vi "PWM2 Set Frequency.vi"(7 "Precision":u16, 9 "Frequency":u32, 10 "ChannelIndex":u8, 11 "DevHandle":i32) -> (3 "function return":i32)   [LabVIEW 2010, in "usb2pwm.lvlib"]
doc: "int WINAPI PWM2_SetFrequency(int DevHandle, unsigned char ChannelIndex, unsigned int Frequency, unsigned short Precision);"
uses:
  usb2pwm.lvlib
  USB2XXX/trunk/USB2XXX/USB2XXX/vs2019/Release/USB2XXX.dll
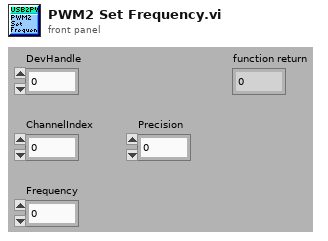
[diagram p1: front panel]
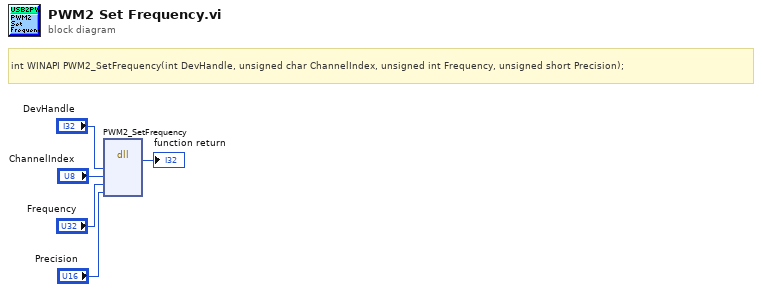
[diagram p0: block diagram]
diagram:
  # "int WINAPI PWM2_SetFrequency(int DevHandle, unsigned char ChannelIndex, unsigned int Frequency, unsigned short Precision);"
  n1 = dll-call lib="E:/Projects/USB2XXX/trunk/USB2XXX/USB2XXX/vs2019/Release/USB2XXX.*" fn="PWM2_SetFrequency"("DevHandle"="DevHandle", "ChannelIndex"="ChannelIndex", "Frequency"="Frequency", "Precision"="Precision") -> (→"function return":i32)  [unwired: 7 in, 2 out]
